vi "ParseControlMoreData.vi"(9 "data out":string) -> (0 "ref1":sgl, 1 "u2":sgl, 2 "u1":sgl, 3 "Bytes read":i32, 4 "ref2":sgl, 5 "x1":sgl, 6 "x2":sgl, 7 "x5":sgl, 8 "x6":sgl)   [LabVIEW 2009]
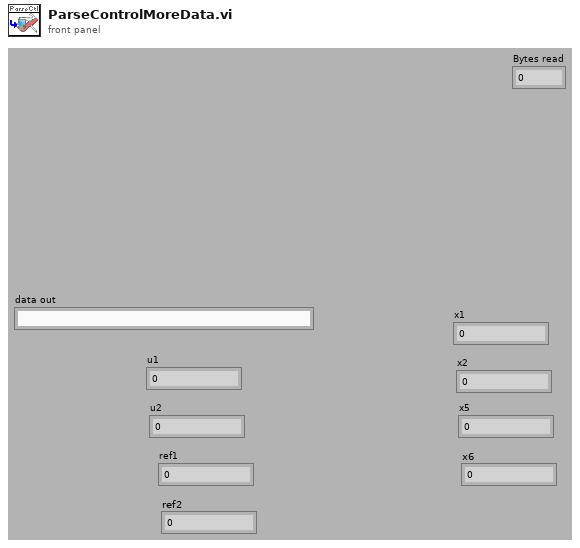
[diagram p1: front panel]
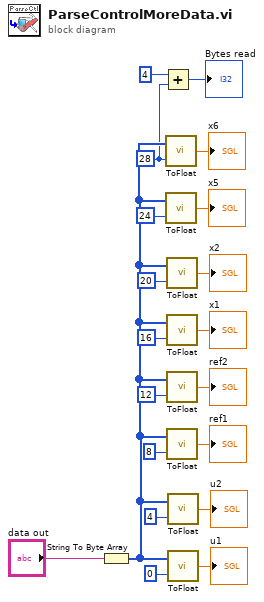
[diagram p0: block diagram]
diagram:
  w1 = 28 ("index")
  n1 = String To Byte Array(string="data out") -> (unsigned byte array=w3:u8[])
  n2 = Add(x=4, y=w1) -> (x+y=→"Bytes read":i32)
  n3 = call "ToFloat.vi"("index"=w1, "array"=w3) -> ("sp float"=→"x6":sgl)
  n4 = call "ToFloat.vi"("index"=24, "array"=w3) -> ("sp float"=→"x5":sgl)
  n5 = call "ToFloat.vi"("index"=20, "array"=w3) -> ("sp float"=→"x2":sgl)
  n6 = call "ToFloat.vi"("index"=16, "array"=w3) -> ("sp float"=→"x1":sgl)
  n7 = call "ToFloat.vi"("index"=12, "array"=w3) -> ("sp float"=→"ref2":sgl)
  n8 = call "ToFloat.vi"("index"=8, "array"=w3) -> ("sp float"=→"ref1":sgl)
  n9 = call "ToFloat.vi"("index"=4, "array"=w3) -> ("sp float"=→"u2":sgl)
  n10 = call "ToFloat.vi"("index"=0, "array"=w3) -> ("sp float"=→"u1":sgl)
